vi "Read Measurement.vi"(8 "error in (no error)":errorcluster, 11 "VISA resource name":refnum<visa-resource-name>) -> (0 "error out":errorcluster, 1 "Units":string, 2 "Weight Value":dbl format="%.3g", 3 "VISA resource name out":refnum<visa-resource-name>, 4 "Stable?":bool, 5 "NET":bool)   [LabVIEW 2015, in "Ohaus AV Series.lvlib"]
doc: "This VI returns the current net weight."
uses:
  Ohaus AV Series.lvlib
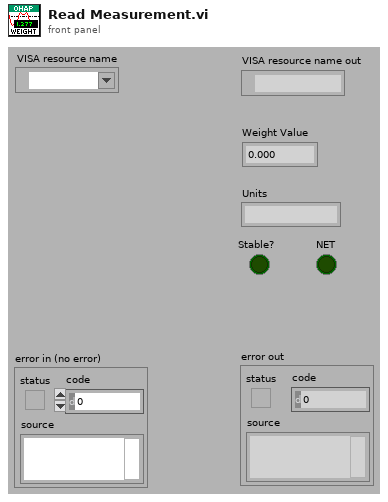
[diagram p1: front panel]
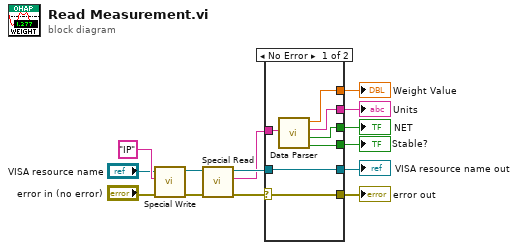
[diagram p0: block diagram]
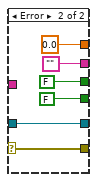
[diagram p2: hidden frame]
diagram:
  n1 = call "Special Write.vi"("error in (no error)"="error in (no error)", "Input String"="IP", "VISA resource name"="VISA resource name") -> ("error out"=w8:errorcluster, "VISA resource name out"=w9:refnum<visa-resource-name>)  [unwired: 7 in]
  n2 = call "Special Read.vi"("error in (no error)"=w8, "VISA resource name"=w9) -> ("error out"=w12:errorcluster, "Output String"=w13:string, "VISA resource name out"=w14:refnum<visa-resource-name>)  [unwired: 7 in]
  n3 = case shown="No Error" w12 {
    selector: w12 -> [w20 w25]
    tunnel: w14 -> [w19 w24]
    tunnel: w13 -> [w21 _]
    tunnel: [w20 w25] -> w11
    tunnel: [w19 w24] -> w10
    tunnel: [w18 "" ("Units")] -> w6
    tunnel: [w17 FALSE ("NET")] -> w5
    tunnel: [w16 FALSE ("Stable?")] -> w4
    tunnel: [w15 0.0 ("Value")] -> w1
    frame No Error {
      n4 = call "Data Parser.vi"("String"=w21) -> ("Stable?"=w16:bool, "NET"=w17:bool, "Units"=w18:string, "Value"=w15:dbl)  [unwired: 7 in]
    }
    frame Error {
    }
  }
  "error out" <- w11
  "VISA resource name out" <- w10
  "Units" <- w6
  "NET" <- w5
  "Stable?" <- w4
  "Weight Value" <- w1
